vi "Lab_Launcher.vi"   [LabVIEW 2020]
panel:
  # "Launches multiple concurrent Diode and Rosie control panels.\nCustomize this VI to match your lab setup."
  # "(See back panel for content)"
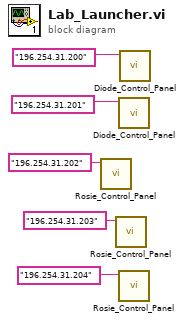
[diagram p0: block diagram]
diagram:
  n1 = call "Rosie_Control_Panel.vi"("IP Address of Remote Device"="196.254.31.202") -> ()  [unwired: 11 in]
  n2 = call "Rosie_Control_Panel.vi"("IP Address of Remote Device"="196.254.31.203") -> ()  [unwired: 11 in]
  n3 = call "Diode_Control_Panel.vi"("IP Address of Remote Device"="196.254.31.201") -> ()  [unwired: 11 in]
  n4 = call "Rosie_Control_Panel.vi"("IP Address of Remote Device"="196.254.31.204") -> ()  [unwired: 11 in]
  n5 = call "Diode_Control_Panel.vi"("IP Address of Remote Device"="196.254.31.200") -> ()  [unwired: 11 in]
